vi "认识布尔.vi"() -> ()   [LabVIEW 2018]
panel:
  in  "停止":bool
  out "或灯":bool
  out "与灯":bool
  in  "布尔 4":bool
  in  "布尔 3":bool
  out "布尔 2":bool
  out "字符串":string="注意开关的机械动作（右键）"
  in  "布尔":bool
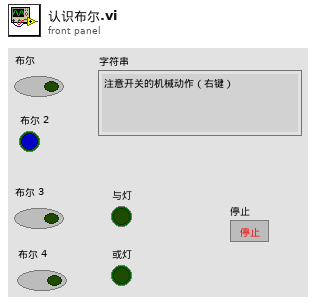
[diagram p1: front panel]
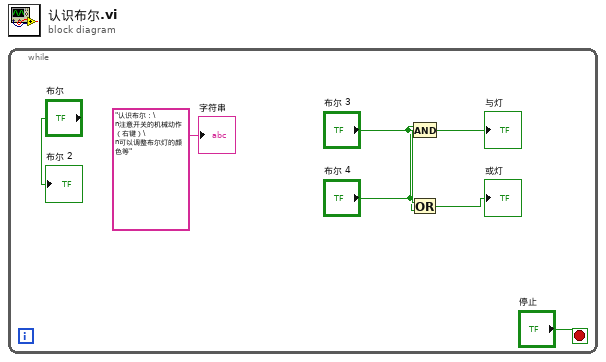
[diagram p0: block diagram]
diagram:
  n1 = while {
    stop <- "停止" stop-if-true
    n2 = And(x="布尔 3", y="布尔 4") -> (x .and. y?=→"与灯":bool)
    n3 = Or(x="布尔 3", y="布尔 4") -> (x .or. y?=→"或灯":bool)
    "字符串" <- "认识布尔：\n注意开关的机械动作（右键）\n可以调整布尔灯的颜色等"
    "布尔 2" <- "布尔"
  }
